vi "1D Look-Up Table (DBL).vi"(2 "LUT":dbl[](array[numeric]) format="%.2f", 3 "index":dbl=0.1 format="%.2f") -> (1 "output point":dbl format="%.2f")   [LabVIEW 2017, in "NI_AdvCtrl_nonlinear.lvlib"]
doc: "LabVIEW no longer supports this VI. You can obtain similar functionality by installing the LabVIEW Simulation Module.\n\nSearches for an element in a given 1D list that has a fractional index (interpolation)."
uses:
  <vilib>/addons/control/advanced/NI_AdvCtrl_nonlinear.lvlib
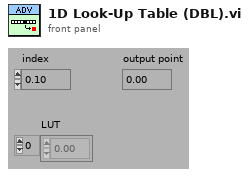
[diagram p1: front panel]
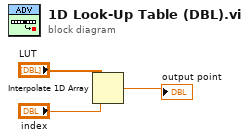
[diagram p0: block diagram]
diagram:
  n1 = Interpolate 1D Array(1:"index", 2:"LUT") -> (0:→"output point":dbl)
